vi "Load Configured Instrument List.vi"(8 "error in (no error)":errorcluster, 11 "Configuration Editor in":refnum<class "Configuration Editor.lvclass">) -> (0 "error out":errorcluster, 3 "Configuration Editor out":refnum<class "Configuration Editor.lvclass">)   [LabVIEW 2023, in "Configuration Editor.lvlib" / "Configuration Editor.lvclass"]
uses:
  Library/Configuration Editor.lvclass
  Library/Configuration Editor.lvclass/Configuration Editor.ctl
  builds/Framework/Configuration.lvlibp/Library/Configuration.lvclass
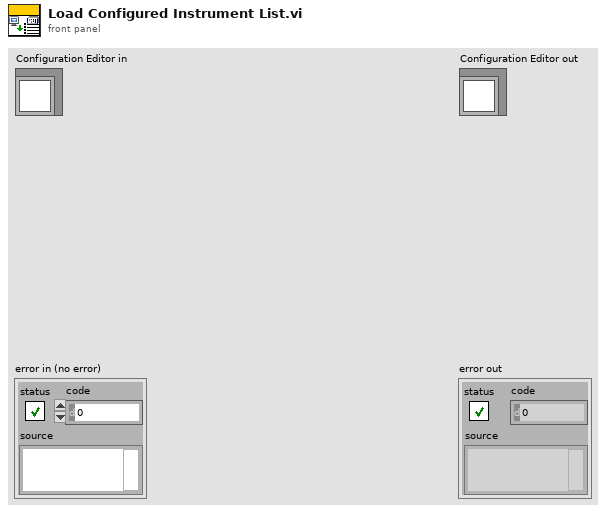
[diagram p1: front panel]
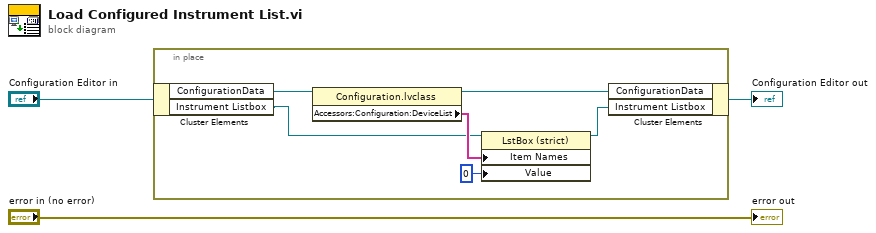
[diagram p0: block diagram]
diagram:
  n1 = in-place {
    n2 = in-place-cluster #1("Configuration Editor in") -> ("ConfigurationData"=w9:refnum<class "Configuration.lvclass">, "Instrument Listbox"=w6:refnum<vi>)
    n3 = property class="Configuration.lvclass"(reference=w9) -> (reference out=w8:refnum<class "Configuration.lvclass">, "Accessors:Configuration:DeviceList"=w7:string[])  [unwired: 1 in, 1 out]
    n4 = property class="LstBox (strict)"(reference=w6, "Item Names"=w7, "Value"=0) -> (reference out=w5:refnum<vi>)  [unwired: 1 in, 1 out]
    n5 = in-place-cluster #1("ConfigurationData"=w8, "Instrument Listbox"=w5) -> (→"Configuration Editor out":refnum<class "Configuration Editor.lvclass">)
  }
  "error out" <- "error in (no error)"
